vi "Get and Set FP Property.vi"(7 "Mode":enum16{"Read", "Write"}(ring), 8 "错误输入（无错误）":errorcluster, 9 "Enable":bool, 10 "Select":T1(ring), 11 "VI Ref In":refnum<vi>) -> (0 "错误输出":errorcluster, 2 "Enable?":bool, 3 "VI Ref Out":refnum<vi>)   [LabVIEW 2012, in "VIRef.lvlib"]
uses:
  VIRef.lvlib
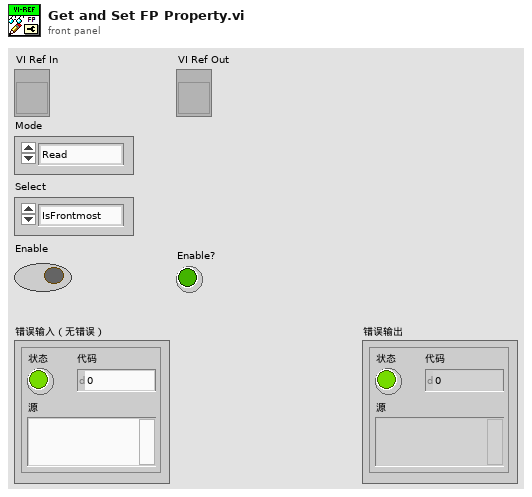
[diagram p1: front panel]
types:
  T1 = enum16{"IsFrontmost", "KeepWinProps", "CustomTile", "Closeable", "Mininmizable", "ShowMenuBar", "HiliteReturnButton", "AllowRTPoup", "TitleBarVis", "Resizeable"}
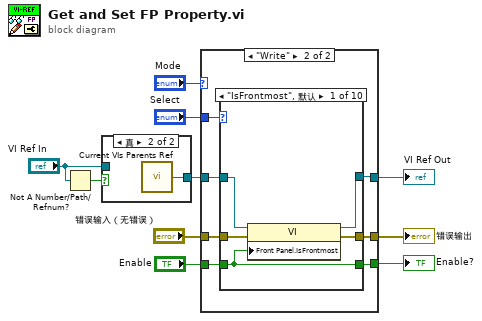
[diagram p0: block diagram]
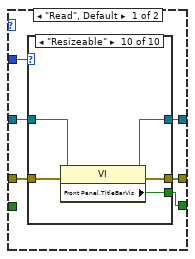
[diagram p2: hidden frame]
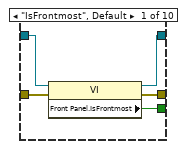
[diagram p3: hidden frame]
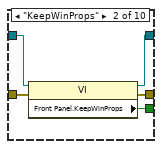
[diagram p4: hidden frame]
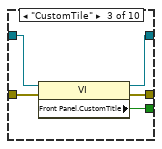
[diagram p5: hidden frame]
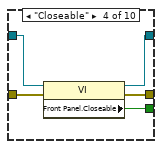
[diagram p6: hidden frame]
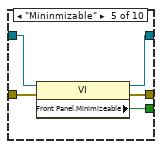
[diagram p7: hidden frame]
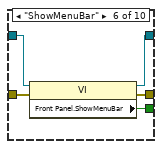
[diagram p8: hidden frame]
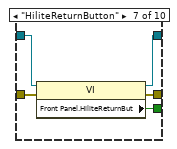
[diagram p9: hidden frame]
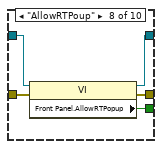
[diagram p10: hidden frame]
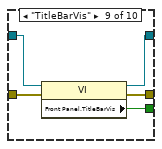
[diagram p11: hidden frame]
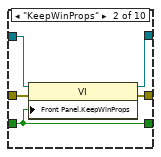
[diagram p12: hidden frame]
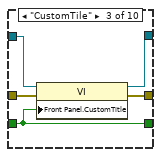
[diagram p13: hidden frame]
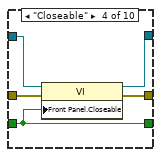
[diagram p14: hidden frame]
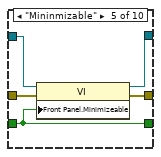
[diagram p15: hidden frame]
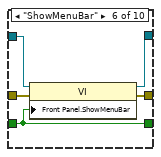
[diagram p16: hidden frame]
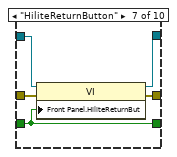
[diagram p17: hidden frame]
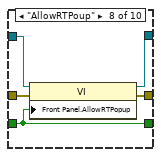
[diagram p18: hidden frame]
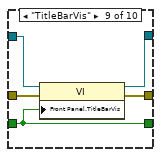
[diagram p19: hidden frame]
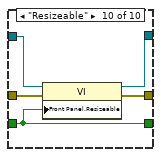
[diagram p20: hidden frame]
diagram:
  n1 = Not A Number/Path/Refnum?(number/path/refnum="VI Ref In") -> (NaN/Path/Refnum?=w10:bool)
  n2 = case shown="真" w10 {
    tunnel: [w11 w12] -> w5
    tunnel: "VI Ref In" -> [w11 _]
    frame False {
    }
    frame True {
      n3 = call "Current VIs Parents Ref.vi"() -> ("Calling VI's Reference"=w12:refnum<vi>)  [unwired: 2 in]
    }
  }
  n4 = case shown="\"Write\"" "Mode" {
    tunnel: "Select" -> [w18 w69]
    tunnel: [w17 w70] -> w6
    tunnel: w5 -> [w16 w74]
    tunnel: "错误输入（无错误）" -> [w15 w75]
    tunnel: [w14 w71] -> w3
    tunnel: [w13 w72] -> w2
    tunnel: "Enable" -> [_ w73]
    frame "Read", Default {
      n5 = case shown="\"Resizeable\"" w18 {
        tunnel: [w21 w28 w31 w34 w39 w44 w49 w54 w59 w65] -> w17
        tunnel: w16 -> [w23 w27 w33 w38 w43 w48 w53 w58 w63 w67]
        tunnel: w15 -> [w22 w26 w32 w36 w42 w47 w51 w57 w62 w66]
        tunnel: [w20 w25 w30 w35 w40 w45 w50 w55 w61 w64] -> w14
        tunnel: [w19 w24 w29 w37 w41 w46 w52 w56 w60 w68] -> w13
        frame "IsFrontmost", Default {
          n6 = property class="VI"(reference=w23, error in=w22) -> (reference out=w19:refnum<vi>, error out=w20:errorcluster, "Front Panel.IsFrontmost"=w21:bool)
        }
        frame "KeepWinProps" {
          n7 = property class="VI"(reference=w27, error in=w26) -> (reference out=w24:refnum<vi>, error out=w25:errorcluster, "Front Panel.KeepWinProps"=w28:bool)
        }
        frame "CustomTile" {
          n8 = property class="VI"(reference=w33, error in=w32) -> (reference out=w29:refnum<vi>, error out=w30:errorcluster, "Front Panel.CustomTitle"=w31:bool)
        }
        frame "Closeable" {
          n9 = property class="VI"(reference=w38, error in=w36) -> (reference out=w37:refnum<vi>, error out=w35:errorcluster, "Front Panel.Closeable"=w34:bool)
        }
        frame "Mininmizable" {
          n10 = property class="VI"(reference=w43, error in=w42) -> (reference out=w41:refnum<vi>, error out=w40:errorcluster, "Front Panel.Minimizeable"=w39:bool)
        }
        frame "ShowMenuBar" {
          n11 = property class="VI"(reference=w48, error in=w47) -> (reference out=w46:refnum<vi>, error out=w45:errorcluster, "Front Panel.ShowMenuBar"=w44:bool)
        }
        frame "HiliteReturnButton" {
          n12 = property class="VI"(reference=w53, error in=w51) -> (reference out=w52:refnum<vi>, error out=w50:errorcluster, "Front Panel.HiliteReturnBut"=w49:bool)
        }
        frame "AllowRTPoup" {
          n13 = property class="VI"(reference=w58, error in=w57) -> (reference out=w56:refnum<vi>, error out=w55:errorcluster, "Front Panel.AllowRTPopup"=w54:bool)
        }
        frame "TitleBarVis" {
          n14 = property class="VI"(reference=w63, error in=w62) -> (reference out=w60:refnum<vi>, error out=w61:errorcluster, "Front Panel.TitleBarVis"=w59:bool)
        }
        frame "Resizeable" {
          n15 = property class="VI"(reference=w67, error in=w66) -> (reference out=w68:refnum<vi>, error out=w64:errorcluster, "Front Panel.TitleBarVis"=w65:bool)
        }
      }
    }
    frame "Write" {
      n16 = case shown="\"IsFrontmost\", 默认" w69 {
        tunnel: [w76 w81 w86 w91 w96 w101 w106 w111 w116 w121] -> w70
        tunnel: [w80 w85 w90 w94 w99 w104 w109 w114 w120 w122] -> w71
        tunnel: [w79 w84 w89 w95 w100 w105 w110 w115 w119 w124] -> w72
        tunnel: w75 -> [w78 w82 w87 w92 w98 w102 w108 w112 w117 w123]
        tunnel: w74 -> [w77 w83 w88 w93 w97 w103 w107 w113 w118 w125]
        tunnel: w73 -> [w76 w81 w86 w91 w96 w101 w106 w111 w116 w121]
        frame "IsFrontmost", Default {
          n17 = property class="VI"(reference=w77, error in=w78, "Front Panel.IsFrontmost"=w76) -> (reference out=w79:refnum<vi>, error out=w80:errorcluster)
        }
        frame "KeepWinProps" {
          n18 = property class="VI"(reference=w83, error in=w82, "Front Panel.KeepWinProps"=w81) -> (reference out=w84:refnum<vi>, error out=w85:errorcluster)
        }
        frame "CustomTile" {
          n19 = property class="VI"(reference=w88, error in=w87, "Front Panel.CustomTitle"=w86) -> (reference out=w89:refnum<vi>, error out=w90:errorcluster)
        }
        frame "Closeable" {
          n20 = property class="VI"(reference=w93, error in=w92, "Front Panel.Closeable"=w91) -> (reference out=w95:refnum<vi>, error out=w94:errorcluster)
        }
        frame "Mininmizable" {
          n21 = property class="VI"(reference=w97, error in=w98, "Front Panel.Minimizeable"=w96) -> (reference out=w100:refnum<vi>, error out=w99:errorcluster)
        }
        frame "ShowMenuBar" {
          n22 = property class="VI"(reference=w103, error in=w102, "Front Panel.ShowMenuBar"=w101) -> (reference out=w105:refnum<vi>, error out=w104:errorcluster)
        }
        frame "HiliteReturnButton" {
          n23 = property class="VI"(reference=w107, error in=w108, "Front Panel.HiliteReturnBut"=w106) -> (reference out=w110:refnum<vi>, error out=w109:errorcluster)
        }
        frame "AllowRTPoup" {
          n24 = property class="VI"(reference=w113, error in=w112, "Front Panel.AllowRTPopup"=w111) -> (reference out=w115:refnum<vi>, error out=w114:errorcluster)
        }
        frame "TitleBarVis" {
          n25 = property class="VI"(reference=w118, error in=w117, "Front Panel.TitleBarVis"=w116) -> (reference out=w119:refnum<vi>, error out=w120:errorcluster)
        }
        frame "Resizeable" {
          n26 = property class="VI"(reference=w125, error in=w123, "Front Panel.Resizeable"=w121) -> (reference out=w124:refnum<vi>, error out=w122:errorcluster)
        }
      }
    }
  }
  "错误输出" <- w3
  "VI Ref Out" <- w2
  "Enable?" <- w6
